vi "Check valid stack ID.vi"(6 "Is real run?":bool, 8 "error in (no error)":errorcluster, 11 "Stack in":refnum<class "Stack.lvclass">) -> (0 "error out":errorcluster, 1 "Non-empty part IDs?":bool, 2 "Valid module ID?":bool, 3 "Stack out":refnum<class "Stack.lvclass">, 4 "Continue with current parts":bool, 5 "Non-empty assembly tray ID?":bool, 7 "Sensor ID out":string)   [LabVIEW 2021, in "Stack.lvclass"]
uses:
  Stack.lvclass
  Stack.lvclass/Stack.ctl
  Assembly/Database Entry/Database Entry.lvclass
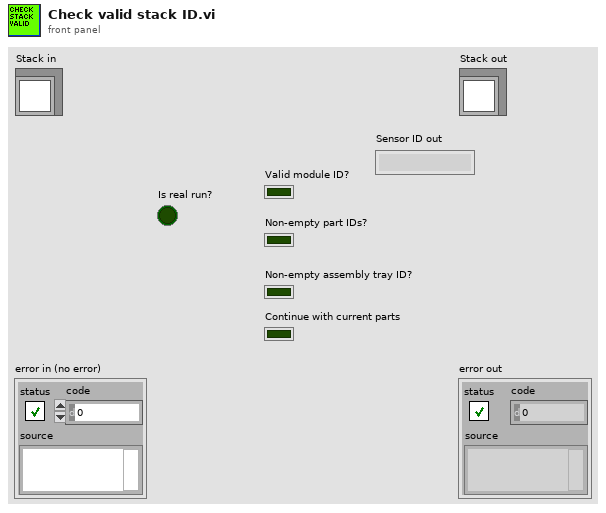
[diagram p1: front panel]
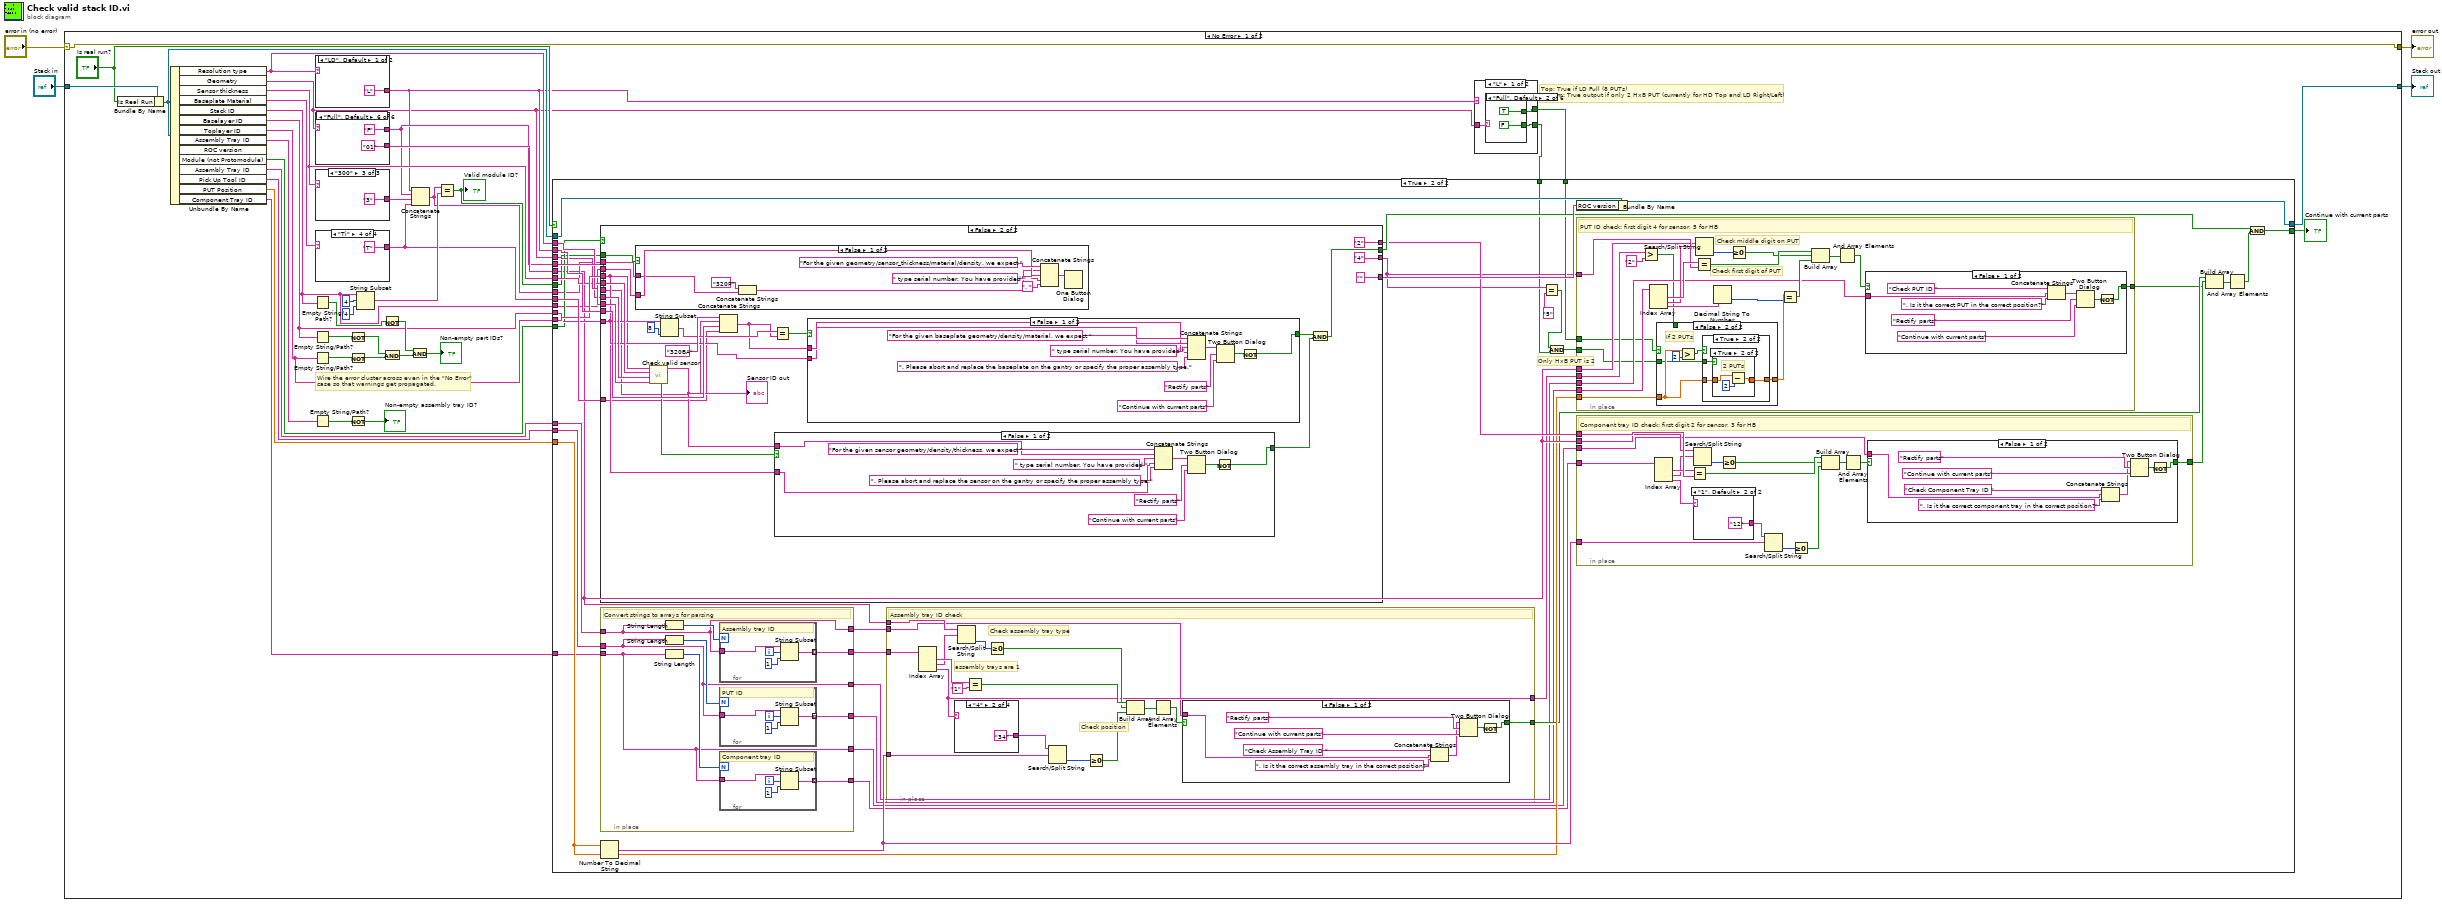
[diagram p0: block diagram]
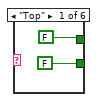
[diagram p2: hidden frame]
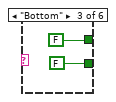
[diagram p3: hidden frame]
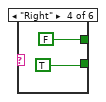
[diagram p4: hidden frame]
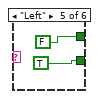
[diagram p5: hidden frame]
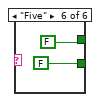
[diagram p6: hidden frame]
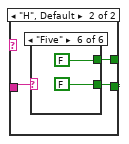
[diagram p7: hidden frame]
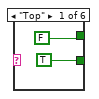
[diagram p8: hidden frame]
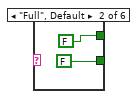
[diagram p9: hidden frame]
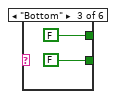
[diagram p10: hidden frame]
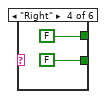
[diagram p11: hidden frame]
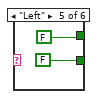
[diagram p12: hidden frame]
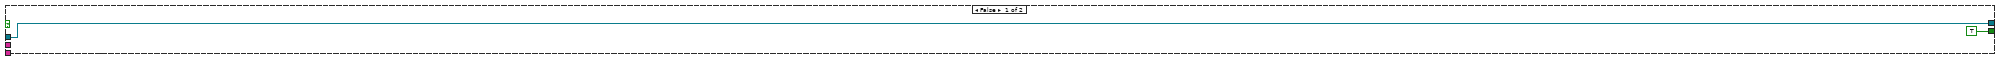
[diagram p13: hidden frame]
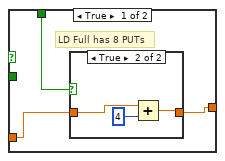
[diagram p14: hidden frame]
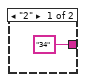
[diagram p19: hidden frame]
diagram:
  n1 = case shown="No Error" "error in (no error)" {
    selector: "error in (no error)" -> [w45 w388]
    tunnel: [w45 w388] -> w3
    tunnel: [w21 w387] -> w1
    tunnel: "Stack in" -> [w28 w387]
    frame No Error {
      # "Top: True if LD Full (8 PUTs)\nBottom: True output if only 2 HxB PUT (currently for HD Top and LD Right/Left)"
      # "Wire the error cluster across even in the \"No Error\"\ncase so that warnings get propagated."
      n2 = Bundle By Name(cluster=w28, "Is Real Run"="Is real run?") -> (w27:refnum<class "Stack.lvclass">)
      n3 = Unbundle By Name(w27) -> ("Resolution type"=w24:string, "Geometry"=w5:string, "Sensor thickness"=w22:string, "Baseplate Material"=w44:string, "Stack ID"=w19:string, "Baselayer ID"=w23:string, "Toplayer ID"=w25:string, "Assembly Tray ID"=w33:string, "Module (not Protomodule)"=w20:bool, "Assembly Tray ID"=w12:string, "Pick Up Tool ID"=w10:string, "PUT Position"=w13:dbl, "Component Tray ID"=w11:string)  [unwired: 1 out]
      n4 = Empty String/Path?(string/path=w19) -> (empty?=w32:bool)
      n5 = Empty String/Path?(string/path=w23) -> (empty?=w39:bool)
      n6 = Empty String/Path?(string/path=w25) -> (empty?=w38:bool)
      n7 = Empty String/Path?(string/path=w33) -> (empty?=w35:bool)
      n8 = case shown="\"LD\", Default" w24 {
        tunnel: ["L" "H"] -> w8
        frame "LD", Default {
        }
        frame "HD" {
        }
      }
      n9 = case shown="\"Full\", Default" w5 {
        tunnel: ["T" "B" "L" "R" "5" "F"] -> w9
        tunnel: ["45" "45" "3" "3" "02" "01"] -> w14
        frame "Top" {
        }
        frame "Bottom" {
        }
        frame "Left" {
        }
        frame "Right" {
        }
        frame "Five" {
        }
        frame "Full", Default {
        }
      }
      n10 = case shown="\"300\"" w22 {
        tunnel: ["2" "1" "3"] -> w43
        frame "200", Default {
        }
        frame "120" {
        }
        frame "300" {
        }
      }
      n11 = case shown="\"Ti\"" w44 {
        tunnel: ["P" "C" "W" "T"] -> w26
        frame "PCB" {
        }
        frame "CF", Default {
        }
        frame "CuW" {
        }
        frame "Ti" {
        }
      }
      n12 = Not(x=w39) -> (.not. x?=w36:bool)
      n13 = Not(x=w38) -> (.not. x?=w37:bool)
      n14 = Not(x=w35) -> (.not. x?=→"Non-empty assembly tray ID?":bool)
      n15 = String Subset(string=w19, offset (0)=4, length (rest)=4 ("length (rest)")) -> (substring=w40:string)
      n16 = Not(x=w32) -> (.not. x?=w31:bool)
      n17 = And(x=w36, y=w37) -> (x .and. y?=w30:bool)
      n18 = And(x=w31, y=w30) -> (x .and. y?=→"Non-empty part IDs?":bool)
      n19 = Concatenate Strings(w8, w9, w43, w26) -> (w18:string)
      n20 = Equal?(x=w18, y=w40) -> (x = y?=w17:bool)
      "Valid module ID?" <- w17
      n21 = case shown="\"L\"" w8 {
        tunnel: w5 -> [w48 w63]
        tunnel: [w47 w62] -> w7
        tunnel: [w46 w61] -> w6
        frame "L" {
          n22 = case shown="\"Full\", Default" w48 {
            tunnel: [FALSE FALSE FALSE TRUE TRUE FALSE] -> w47
            tunnel: [FALSE TRUE FALSE FALSE FALSE FALSE] -> w46
            frame "Top" {
            }
            frame "Full", Default {
            }
            frame "Bottom" {
            }
            frame "Right" {
            }
            frame "Left" {
            }
            frame "Five" {
            }
          }
        }
        frame "H", Default {
          n23 = case shown="\"Five\"" w63 {
            tunnel: [TRUE FALSE FALSE FALSE FALSE FALSE] -> w62
            tunnel: [FALSE FALSE FALSE FALSE FALSE FALSE] -> w61
            frame "Top" {
            }
            frame "Full", Default {
            }
            frame "Bottom" {
            }
            frame "Right" {
            }
            frame "Left" {
            }
            frame "Five" {
            }
          }
        }
      }
      n24 = case shown="True" "Is real run?" {
        tunnel: w27 -> [w76 w84]
        tunnel: w9 -> [_ w119]
        tunnel: w8 -> [_ w118]
        tunnel: w26 -> [_ w117]
        tunnel: w25 -> [_ w116]
        tunnel: w5 -> [_ w115]
        tunnel: w24 -> [_ w114]
        tunnel: w23 -> [_ w113]
        tunnel: w22 -> [_ w112]
        tunnel: [w76 w111] -> w21
        tunnel: w20 -> [_ w109]
        tunnel: w19 -> [_ w108]
        tunnel: w18 -> [_ w107]
        tunnel: w17 -> [_ w106]
        tunnel: [TRUE w104] -> w16
        tunnel: w14 -> [_ w101]
        tunnel: w13 -> [_ w100]
        tunnel: w12 -> [_ w93]
        tunnel: w11 -> [_ w92]
        tunnel: w10 -> [_ w91]
        tunnel: w7 -> [_ w78]
        tunnel: w6 -> [_ w83]
        frame False {
        }
        frame True {
          # "Only HxB PUT is 2"
          n25 = case shown="False" w109 {
            tunnel: w119 -> [w270 w316]
            tunnel: w118 -> [w271 w335]
            tunnel: w117 -> [_ w318]
            tunnel: w116 -> [w267 w323]
            tunnel: w115 -> [_ w329]
            tunnel: w112 -> [_ w328]
            tunnel: w114 -> [_ w327]
            tunnel: w113 -> [w266 w324]
            tunnel: [w260 w320] -> w105
            tunnel: [w255 "" ("String")] -> w110
            tunnel: w108 -> [w254 w317]
            tunnel: w107 -> [w252 w315]
            tunnel: w106 -> [w253 w314]
            tunnel: ["3" ("y") "2" ("y")] -> w103
            tunnel: ["5" ("y") "4" ("y")] -> w81
            frame True {
              w257 = path "roc_version.csv" ("name or relative path")
              # "Using 'not' in the Yes/No box is deliberate. \nWant the default to be rectify parts"
              n26 = case shown="False" w253 {
                tunnel: w254 -> [w280 _]
                tunnel: w252 -> [w279 _]
                frame False {
                  n27 = Concatenate Strings("320M" ("string"), w279) -> (w278:string)
                  n28 = Concatenate Strings("For the given geometry/sensor_thickness/material/density, we expect " ("message"), w278, " type serial number. You have provided " ("string"), w280, ". " ("string")) -> (w281:string)
                  n29 = One Button Dialog(message=w281) -> ()  [unwired: 1 in, 1 out]
                }
                frame True {
                }
              }
              n30 = String Subset(string=w267, length (rest)=6 ("length (rest)")) -> (substring=w275:string)  [unwired: 1 in]
              n31 = String Subset(string=w267, offset (0)=7, length (rest)=1 ("length (rest)")) -> (substring=w259:string)
              n32 = String Subset(string=w266, offset (0)=8, length (rest)=1 ("length (rest)")) -> (substring=w256:string)
              n33 = Concatenate Strings("320X" ("string"), w271, w270) -> (w274:string)
              n34 = Equal?(x=w275, y=w274) -> (x = y?=w273:bool)
              n35 = Equal?(x=w259, y=w256) -> (x = y?=w263:bool)
              n36 = call "Get kind of part.vi"("Element"=w259, "File Path"=w257) -> ("Element definiton out"=w258:string)  [unwired: 9 in]
              n37 = call "Get kind of part.vi"("Element"=w256, "File Path"=w257) -> ("Element definiton out"=w255:string)  [unwired: 9 in]
              n38 = case shown="False" w273 {
                tunnel: w274 -> [w309 _]
                tunnel: w267 -> [w305 _]
                tunnel: [w303 TRUE] -> w262
                frame False {
                  n39 = Concatenate Strings("For the given hexaboard geometry/density, we expect " ("message"), w309, " type serial number. You have provided " ("string"), w305, ". Please abort and replace the hexaboard on the gantry or specify the proper assembly type." ("string")) -> (w307:string)
                  n40 = Two Button Dialog(message=w307, 1:"Continue with current parts" ("T button name (\"OK\")"), 2:"Rectify parts" ("F button name (\"Cancel\")")) -> (T button?=w304:bool)
                  n41 = Not(x=w304) -> (.not. x?=w303:bool)
                }
                frame True {
                }
              }
              n42 = case shown="False" w263 {
                tunnel: w267 -> [w299 _]
                tunnel: w258 -> [w298 _]
                tunnel: w266 -> [w296 _]
                tunnel: w255 -> [w289 _]
                tunnel: [w288 TRUE] -> w261
                frame False {
                  w295 = " is defined as a " ("string")
                  n43 = Concatenate Strings(w299, w295, w298, " hexaboard. " ("string")) -> (w293:string)
                  n44 = Concatenate Strings(w296, w295, w289, " protomodule. " ("string")) -> (w292:string)
                  n45 = Concatenate Strings(w293, w292, "If this is unintended, please replace the hexaboard or rename the protomodule before continuing assembly." ("string")) -> (w290:string)
                  n46 = Two Button Dialog(message=w290, 1:"Continue with current parts" ("T button name (\"OK\")"), 2:"Rectify parts" ("F button name (\"Cancel\")")) -> (T button?=w287:bool)
                  n47 = Not(x=w287) -> (.not. x?=w288:bool)
                }
                frame True {
                }
              }
              n48 = And(x=w262, y=w261) -> (x .and. y?=w260:bool)
            }
            frame False {
              n49 = case shown="False" w314 {
                tunnel: w317 -> [w339 _]
                tunnel: w315 -> [w338 _]
                frame False {
                  n50 = Concatenate Strings("320P" ("string"), w338) -> (w337:string)
                  n51 = Concatenate Strings("For the given geometry/sensor_thickness/material/density, we expect " ("message"), w337, " type serial number. You have provided " ("string"), w339, ". " ("string")) -> (w340:string)
                  n52 = One Button Dialog(message=w340) -> ()  [unwired: 1 in, 1 out]
                }
                frame True {
                }
              }
              n53 = call "Check valid sensor.vi"("Geometry in"=w329, "Resolution in"=w327, "Thickness in"=w328, "Sensor ID"=w323) -> ("Sensor ID out"=w330:string, "Sensor ID okay"=w326:bool)  [unwired: 3 in, 3 out]
              "Sensor ID out" <- w330
              n54 = String Subset(string=w324, length (rest)=8 ("length (rest)")) -> (substring=w332:string)  [unwired: 1 in]
              n55 = Concatenate Strings("320BA" ("string"), w316, w335, w318) -> (w331:string)
              n56 = Equal?(x=w332, y=w331) -> (x = y?=w325:bool)
              n57 = case shown="False" w326 {
                tunnel: w330 -> [w352 _]
                tunnel: w323 -> [w348 _]
                tunnel: [w346 TRUE] -> w321
                frame False {
                  n58 = Concatenate Strings("For the given sensor geometry/density/thickness, we expect " ("message"), w352, " type serial number. You have provided " ("string"), w348, ". Please abort and replace the sensor on the gantry or specify the proper assembly type." ("string")) -> (w350:string)
                  n59 = Two Button Dialog(message=w350, 1:"Continue with current parts" ("T button name (\"OK\")"), 2:"Rectify parts" ("F button name (\"Cancel\")")) -> (T button?=w347:bool)
                  n60 = Not(x=w347) -> (.not. x?=w346:bool)
                }
                frame True {
                }
              }
              n61 = case shown="False" w325 {
                tunnel: w331 -> [w363 _]
                tunnel: w324 -> [w359 _]
                tunnel: [w357 TRUE] -> w322
                frame False {
                  n62 = Concatenate Strings("For the given baseplate geometry/density/material, we expect " ("message"), w363, " type serial number. You have provided " ("string"), w359, ". Please abort and replace the baseplate on the gantry or specify the proper assembly type." ("string")) -> (w361:string)
                  n63 = Two Button Dialog(message=w361, 1:"Continue with current parts" ("T button name (\"OK\")"), 2:"Rectify parts" ("F button name (\"Cancel\")")) -> (T button?=w358:bool)
                  n64 = Not(x=w358) -> (.not. x?=w357:bool)
                }
                frame True {
                }
              }
              n65 = And(x=w322, y=w321) -> (x .and. y?=w320:bool)
            }
          }
          n66 = in-place {
            in-place-border: w93 -> [w120]
            in-place-border: [w127] -> w90
            in-place-border: w92 -> [w121]
            in-place-border: [w125] -> w89
            in-place-border: w91 -> [w122]
            in-place-border: [w123] -> w88
            in-place-border: [w122] -> w87
            in-place-border: [w121] -> w86
            in-place-border: [w120] -> w85
            # "Convert strings to arrays for parsing"
            n67 = String Length(string=w120) -> (length=w128:i32)
            n68 = String Length(string=w122) -> (length=w124:i32)
            n69 = String Length(string=w121) -> (length=w126:i32)
            n70 = for {
              N: w128 -> [_]
              tunnel: w120 -> [w140]
              tunnel: [w137] -> w127 mode=indexing
              i -> [w138]
              # "Assembly tray ID"
              n71 = String Subset(string=w140, offset (0)=w138, length (rest)=1 ("length (rest)")) -> (substring=w137:string)
            }
            n72 = for {
              N: w124 -> [_]
              tunnel: w122 -> [w132]
              tunnel: [w129] -> w123 mode=indexing
              i -> [w130]
              # "PUT ID"
              n73 = String Subset(string=w132, offset (0)=w130, length (rest)=1 ("length (rest)")) -> (substring=w129:string)
            }
            n74 = for {
              N: w126 -> [_]
              tunnel: w121 -> [w136]
              tunnel: [w133] -> w125 mode=indexing
              i -> [w134]
              # "Component tray ID"
              n75 = String Subset(string=w136, offset (0)=w134, length (rest)=1 ("length (rest)")) -> (substring=w133:string)
            }
          }
          n76 = Number To Decimal String(number=w100) -> (decimal integer string=w102:string)  [unwired: 1 in]
          n77 = in-place {
            in-place-border: w90 -> [w235]
            in-place-border: w101 -> [w223]
            in-place-border: [w231] -> w98
            in-place-border: w102 -> [w222]
            in-place-border: [w221] -> w99
            in-place-border: w85 -> [w220]
            # "Check position"
            # "Check assembly tray type"
            # "assembly trays are 1"
            # "Assembly tray ID check"
            n78 = Index Array(array=w235) -> (element #1=w234:string, element #2=w232:string, element #3=w221:string)  [unwired: 3 in]
            n79 = case shown="\"4\"" w221 {
              tunnel: ["34" ("string") "34" ("string") "12" ("string") "12" ("string")] -> w230
              frame "2" {
              }
              frame "4" {
              }
              frame "1", Default {
              }
              frame "3" {
              }
            }
            n80 = Search/Split String(string=w223, search string/char (-)=w232) -> (offset of match=w233:i32)  [unwired: 1 in, 2 out]
            n81 = Equal?(x=w234, y="1") -> (x = y?=w228:bool)
            n82 = Greater Or Equal To 0?(x=w233) -> (x >= 0?=w227:bool)
            n83 = Search/Split String(string=w230, search string/char (-)=w222) -> (offset of match=w229:i32)  [unwired: 1 in, 2 out]
            n84 = Greater Or Equal To 0?(x=w229) -> (x >= 0?=w226:bool)
            n85 = Build Array(w228, w227, w226) -> (w225:bool[])
            n86 = And Array Elements(Boolean array=w225) -> (logical AND=w224:bool)
            n87 = case shown="False" w224 {
              selector: w224 -> [_ w249]
              tunnel: [w245 w249] -> w231
              tunnel: w220 -> [w241 _]
              frame False {
                n88 = Concatenate Strings("Check Assembly Tray ID " ("string"), w241, ". Is it the correct assembly tray in the correct position?" ("string")) -> (w243:string)
                n89 = Two Button Dialog(message=w243, 1:"Continue with current parts" ("T button name (\"OK\")"), 2:"Rectify parts" ("F button name (\"Cancel\")")) -> (T button?=w246:bool)
                n90 = Not(x=w246) -> (.not. x?=w245:bool)
              }
              frame True {
              }
            }
          }
          n91 = Equal?(x=w81, y="5") -> (x = y?=w80:bool)
          n92 = And(x=w80, y=w78) -> (x .and. y?=w79:bool)
          n93 = Bundle By Name(cluster=w84, "ROC version"=w110) -> (w111:refnum<class "Stack.lvclass">)
          n94 = in-place {
            in-place-border: w88 -> [w162]
            in-place-border: [w160] -> w96
            in-place-border: w81 -> [w153]
            in-place-border: w101 -> [w152]
            in-place-border: w100 -> [w144]
            in-place-border: w99 -> [w150]
            in-place-border: w87 -> [w145]
            in-place-border: w79 -> [w143]
            in-place-border: w83 -> [w142]
            # "Check first digit of PUT"
            # "Check middle digit on PUT"
            # "PUT ID check: first digit 4 for sensor, 5 for HB"
            n95 = Greater?(x=w150, y="2") -> (0:w141:bool)
            n96 = Index Array(array=w162) -> (element #1=w161:string, element #2=w159:string, element #3=w151:string)  [unwired: 3 in]
            n97 = case shown="False" w142 {
              tunnel: [w163 w174] -> w148
              tunnel: w144 -> [w164 w173]
              tunnel: w143 -> [_ w170]
              tunnel: w141 -> [w165 _]
              frame True {
                # "LD Full has 8 PUTs"
                n98 = case shown="True" w165 {
                  tunnel: w164 -> [w166 w168]
                  tunnel: [w166 w169] -> w163
                  frame False {
                  }
                  frame True {
                    n99 = Add(x=w168, y=4) -> (x+y=w169:dbl)
                  }
                }
              }
              frame False {
                # "If 2 PUTs"
                n100 = Greater?(x=w173, y=2) -> (0:w171:bool)
                n101 = case shown="True" w171 {
                  tunnel: w173 -> [w175 w178]
                  tunnel: [w175 w177] -> w174
                  tunnel: w170 -> [_ w176]
                  frame False {
                    # "4 PUTs"
                  }
                  frame True {
                    n102 = case shown="True" w176 {
                      tunnel: w178 -> [w179 w181]
                      tunnel: [w179 w182] -> w177
                      frame False {
                        # "4 PUTs"
                      }
                      frame True {
                        # "2 PUTs"
                        n103 = Subtract(x=w181, y=2) -> (x-y=w182:dbl)
                      }
                    }
                  }
                }
              }
            }
            n104 = Search/Split String(string=w152, search string/char (-)=w159) -> (offset of match=w158:i32)  [unwired: 1 in, 2 out]
            n105 = Equal?(x=w161, y=w153) -> (x = y?=w157:bool)
            n106 = Decimal String To Number(string=w151) -> (number=w147:i32)  [unwired: 2 in, 1 out]
            n107 = Greater Or Equal To 0?(x=w158) -> (x >= 0?=w156:bool)
            n108 = Equal?(x=w148, y=w147) -> (x = y?=w146:bool)
            n109 = Build Array(w157, w156, w146) -> (w155:bool[])
            n110 = And Array Elements(Boolean array=w155) -> (logical AND=w154:bool)
            n111 = case shown="False" w154 {
              selector: w154 -> [_ w191]
              tunnel: [w187 w191] -> w160
              tunnel: w145 -> [w185 _]
              frame False {
                n112 = Concatenate Strings("Check PUT ID " ("string"), w185, ". Is it the correct PUT in the correct position?" ("string")) -> (w183:string)
                n113 = Two Button Dialog(message=w183, 1:"Continue with current parts" ("T button name (\"OK\")"), 2:"Rectify parts" ("F button name (\"Cancel\")")) -> (T button?=w188:bool)
                n114 = Not(x=w188) -> (.not. x?=w187:bool)
              }
              frame True {
              }
            }
          }
          n115 = in-place {
            in-place-border: w89 -> [w208]
            in-place-border: w103 -> [w207]
            in-place-border: [w205] -> w97
            in-place-border: w101 -> [w204]
            in-place-border: w102 -> [w193]
            in-place-border: w86 -> [w192]
            # "Component tray ID check: first digit 2 for sensor, 3 for HB"
            n116 = Index Array(array=w208) -> (element #1=w206:string, element #2=w203:string, element #3=w195:string)  [unwired: 3 in]
            n117 = Equal?(x=w206, y=w207) -> (x = y?=w201:bool)
            n118 = Search/Split String(string=w204, search string/char (-)=w203) -> (offset of match=w202:i32)  [unwired: 1 in, 2 out]
            n119 = case shown="\"1\", Default" w195 {
              tunnel: ["34" ("string") "12" ("string")] -> w197
              frame "2" {
              }
              frame "1", Default {
              }
            }
            n120 = Greater Or Equal To 0?(x=w202) -> (x >= 0?=w200:bool)
            n121 = Search/Split String(string=w197, search string/char (-)=w193) -> (offset of match=w196:i32)  [unwired: 1 in, 2 out]
            n122 = Greater Or Equal To 0?(x=w196) -> (x >= 0?=w194:bool)
            n123 = Build Array(w201, w200, w194) -> (w199:bool[])
            n124 = And Array Elements(Boolean array=w199) -> (logical AND=w198:bool)
            n125 = case shown="False" w198 {
              selector: w198 -> [_ w219]
              tunnel: [w215 w219] -> w205
              tunnel: w192 -> [w213 _]
              frame False {
                n126 = Concatenate Strings("Check Component Tray ID " ("string"), w213, ". Is it the correct component tray in the correct position?" ("string")) -> (w212:string)
                n127 = Two Button Dialog(message=w212, 1:"Continue with current parts" ("T button name (\"OK\")"), 2:"Rectify parts" ("F button name (\"Cancel\")")) -> (T button?=w216:bool)
                n128 = Not(x=w216) -> (.not. x?=w215:bool)
              }
              frame True {
              }
            }
          }
          n129 = Build Array(w98, w97, w96) -> (w95:bool[])
          n130 = And Array Elements(Boolean array=w95) -> (logical AND=w94:bool)
          n131 = And(x=w105, y=w94) -> (x .and. y?=w104:bool)
        }
      }
      "Continue with current parts" <- w16
    }
    frame Error {
    }
  }
  "error out" <- w3
  "Stack out" <- w1
